vi "Do.vi"(8 "error in (no error)":errorcluster, 10 "Actor in":refnum<class "Actor.lvclass">, 11 "New Results Msg":refnum<class "New Results Msg.lvclass">) -> (0 "error out":errorcluster, 2 "Actor out":refnum<class "Actor.lvclass">)   [LabVIEW 2014, in "HIJ Vision Application.lvlib" / "New Results Msg.lvclass"]
doc: "This VI delivers the message to the actor by calling the appropriate method(s) on the actor."
uses:
  New Results Msg.lvclass
  <vilib>/ActorFramework/Actor/Actor.lvclass
  HIJ Vision Application/HIJ Vision Application.lvclass
  Abstract Messages/Publish Analyze Results Msg/Publish Analyze Results Msg.lvclass/Publish Analyze Results Msg.ctl
  Abstract Messages/Publish Analyze Results Msg/Publish Analyze Results Msg.lvclass
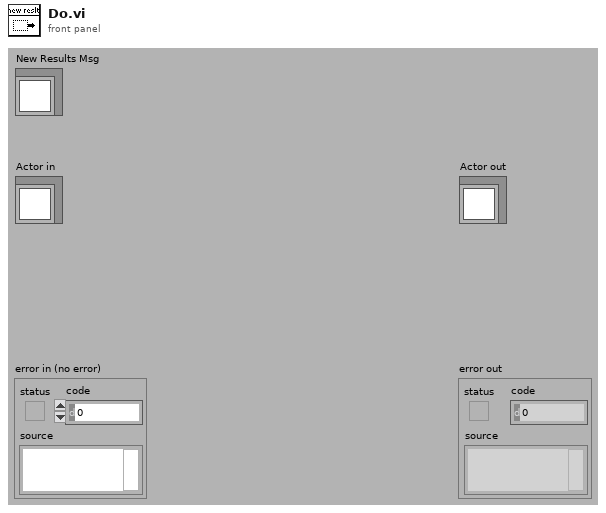
[diagram p1: front panel]
types:
  T1 = cluster{"Image Nr.":i32, "Results":refnum<class "Analyze Results Base.lvclass">[], "Parameters":refnum<class "Analyze Parameter Base.lvclass">[]}
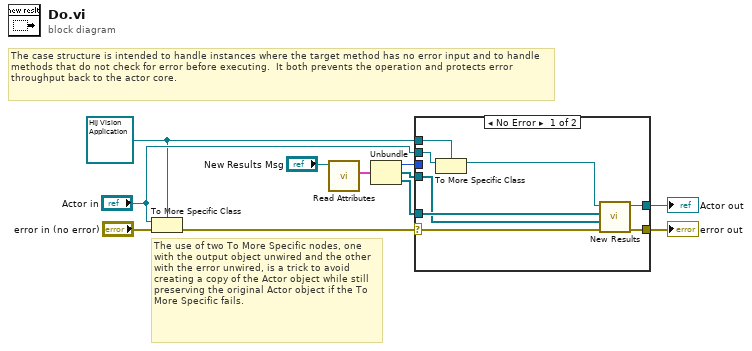
[diagram p0: block diagram]
diagram:
  w6 = refnum<class "HIJ Vision Application.lvclass"> refnum ("Actor in")
  # "The use of two To More Specific nodes, one with the output object unwired and the other with the error unwired, is a trick to avoid creating a copy of the Actor object while still preserving the original Actor object if the To More Specific fails."
  # "The case structure is intended to handle instances where the target method has no error input and to handle methods that do not check for error before executing.  It both prevents the operation and protects error throughput back to the actor core."
  n1 = To More Specific Class(target class=w6, reference="Actor in", error in="error in (no error)") -> (error out=w10:errorcluster)  [unwired: 1 out]
  n2 = call "Read Attributes.vi"("Abstract Message Template in"="New Results Msg") -> ("Payload"=w4:T1)  [unwired: 9 in, 1 out]
  n3 = Unbundle(w4) -> ("Image Nr."=w3:i32, "Results"=w2:refnum<class "Analyze Results Base.lvclass">[], "Parameters"=w1:refnum<class "Analyze Parameter Base.lvclass">[])
  n4 = case shown="No Error" w10 {
    selector: w10 -> [w17 w21]
    tunnel: [w19 w21] -> w9
    tunnel: [w18 w20] -> w8
    tunnel: "Actor in" -> [w16 w20]
    tunnel: w6 -> [w15 _]
    tunnel: w3 -> [_ _]
    tunnel: w2 -> [w12 _]
    tunnel: w1 -> [w13 _]
    frame No Error {
      n5 = To More Specific Class(target class=w15, reference=w16) -> (specific class reference=w14:refnum<class "HIJ Vision Application.lvclass">)  [unwired: 1 in, 1 out]
      n6 = call "New Results.vi"("error in (no error)"=w17, "Results In"=w12, "Parameters"=w13, "Launch IMAQ Display in"=w14) -> ("error out"=w19:errorcluster, "Launch IMAQ Display out"=w18:refnum<class "HIJ Vision Application.lvclass">)  [unwired: 6 in]
    }
    frame Error {
      # "If type check fails, pass the original object out again."
    }
  }
  "error out" <- w9
  "Actor out" <- w8
